vi "Executor.vi"(0 "Future":refnum<class "Future.lvclass">) -> ()   [LabVIEW 2017, in "Promise Future.lvlib" / "Future.lvclass"]
doc: "(<B>Filename</B>: Actor Framework.lvlib:Actor.lvclass:Actor.vi)\n\nActor.vi is the top-level VI that is launched to be the functional aspect of the actor object. It is a wrapper around Actor Core.vi, which is where the actor defines most of its specific behavior. Actor.vi takes care of creating the caller-to-actor queue and brokering the exchange of enqueuers with the caller. It also handles all the cleanup when Actor Core.vi completes. It is not dynamic dispatch -- users of the actor framework generally don't need to understand what's being done in this function."
uses:
  Future.lvclass
  Future.lvclass/Future.ctl
  70fb4332-8571-40f3-8f9a-39d1e70c4e03.vi
  Read Value.vi
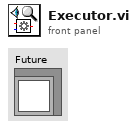
[diagram p1: front panel]
types:
  T1 = typedef "Semaphore RefNum" = refnum<k1>
  T2 = cluster{"type specifier VI Refnum (for type only)":refnum<vi>, "Scope":variant}
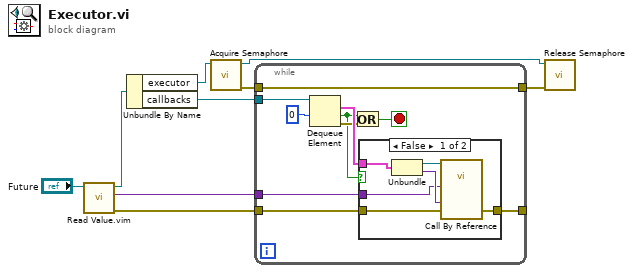
[diagram p0: block diagram]
diagram:
  n1 = call "Read Value.vim"("Future in"="Future") -> ("error out"=w4:errorcluster, "Value"=w3:variant, "Future out"=w5:refnum<class "Future.lvclass">)  [unwired: 7 in, 1 out]
  n2 = Unbundle By Name(w5) -> ("executor"=w1:T1, "callbacks"=w6:refnum<queue>)
  n3 = call <vilib>:"Acquire Semaphore.vi"("semaphore"=w1) -> ("error out"=w8:errorcluster, "semaphore out"=w9:T1)  [unwired: 4 in, 1 out]
  n4 = while {
    tunnel: w6 -> [w19]
    tunnel: w3 -> [w17]
    tunnel: w4 -> [w15]
    tunnel: [w11] -> _
    tunnel: w8 -> [w10]
    tunnel: [w10] -> w7
    stop <- w12 stop-if-true
    n5 = Dequeue Element(queue=w19, timeout in ms (-1)=0) -> (element=w16:T2, timed out?=w13:bool, error out=w14:errorcluster)  [unwired: 1 in, 1 out]
    n6 = Or(x=w13, y=w14) -> (x .or. y?=w12:bool)
    n7 = case shown="False" w13 {
      tunnel: w17 -> [w22 _]
      tunnel: w16 -> [w25 _]
      tunnel: w15 -> [w21 w26]
      tunnel: [w20 w26] -> w11
      frame False {
        n8 = Unbundle(w25) -> ("type specifier VI Refnum (for type only)"=w24:refnum<vi>, "Scope"=w23:variant)
        n9 = call-by-ref "?"(reference=w24, "error in (no error)"=w21, "Scope"=w23, "Value"=w22) -> ("error out"=w20:errorcluster)  [unwired: 9 in, 2 out]
      }
      frame True {
      }
    }
  }
  n10 = call <vilib>:"Release Semaphore.vi"("error in (no error)"=w7, "semaphore"=w9) -> ()  [unwired: 4 in, 2 out]
